vi "Generate Legend Box.vi"(8 "rect 2":T1, 10 "Array Size":i32, 11 "Height":u32) -> (0 "rect":T1, 3 "Gap":i32=30)   [LabVIEW 2016, in "CML UI.lvlib" / "Circular Cue Helper.lvlib"]
doc: "This VI generates the Legend Box of the pie chart"
uses:
  Circular Cue Helper.lvlib
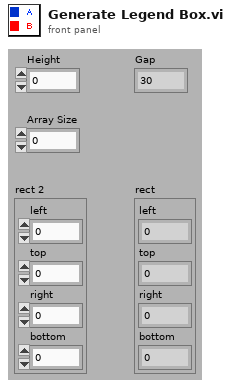
[diagram p1: front panel]
types:
  T1 = cluster{"left":i16, "top":i16, "right":i16, "bottom":i16}
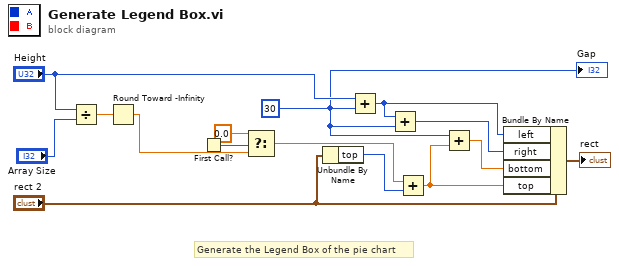
[diagram p0: block diagram]
diagram:
  w1 = 30
  # "Generate the Legend Box of the pie chart"
  n1 = Divide(x="Height", y="Array Size") -> (x/y=w3:dbl)
  n2 = Round Toward -Infinity(1:w3) -> (0:w2:dbl)
  n3 = First Call?() -> (First Call?: T/F=w7:bool)
  n4 = Select(t=0.0, s=w7, f=w2) -> (s? t:f=w6:dbl)
  n5 = Unbundle By Name("rect 2") -> ("top"=w14:i16)
  n6 = Add(x="Height", y=w1) -> (x+y=w11:u32)
  n7 = Add(x=w11, y=w1) -> (x+y=w10:u32)
  n8 = Add(x=w6, y=w14) -> (x+y=w13:dbl)
  n9 = Add(x=w1, y=w13) -> (x+y=w12:dbl)
  n10 = Bundle By Name(cluster="rect 2", "left"=w11, "right"=w10, "bottom"=w12, "top"=w13) -> (→"rect":T1)
  "Gap" <- w1
